vi "State Enter Core.vi"(8 "error in (no error)":errorcluster, 11 "A Context State in":refnum<class "A Context State.lvclass">) -> (0 "error out":errorcluster, 3 "A Context State out":refnum<class "A Context State.lvclass">)   [LabVIEW 2021, in "Context Actor.lvlib" / "A Context State.lvclass"]
uses:
  A Context State.lvclass
  A Context State.lvclass/A Context State.ctl
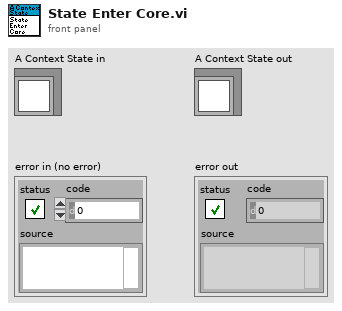
[diagram p1: front panel]
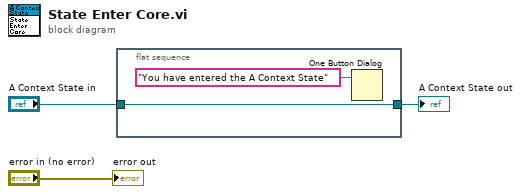
[diagram p0: block diagram]
diagram:
  n1 = flat-sequence {
    tunnel: [w4] -> w2
    tunnel: "A Context State in" -> [w4]
    frame #0 {
      n2 = One Button Dialog(message="You have entered the A Context State") -> ()  [unwired: 1 in, 1 out]
    }
  }
  "error out" <- "error in (no error)"
  "A Context State out" <- w2
